vi "Snippets.vi"(6 "args":string[](array[string]), 7 "QD Plugins Dir":path, 8 "error in (no error)":errorcluster, 9 "Shift?":bool, 10 "Focus":enum8{"FP", "BD"}(ring), 11 "VI Refnum":refnum<vi>) -> (0 "error out":errorcluster)   [LabVIEW 2019]
doc: "Imports or exports a VI Snippet (*.png) image programmatically. Import opens a preview dialog to select a VI Snippet (*.png) from the <b>QuickDrop\\plugins\\Snippets</b> directory. Export prompts the user where to save the VI Snippet (*.png). On export, if nothing is selected the entire VI is exported. Otherwise only the selected Block Diagram GObjects are exported.\n\n[SCRIPT]\nimport=Import VI Snippet\nexport=Export VI Snippet"
uses:
  _Snippets/VI Snippet.lvlibp
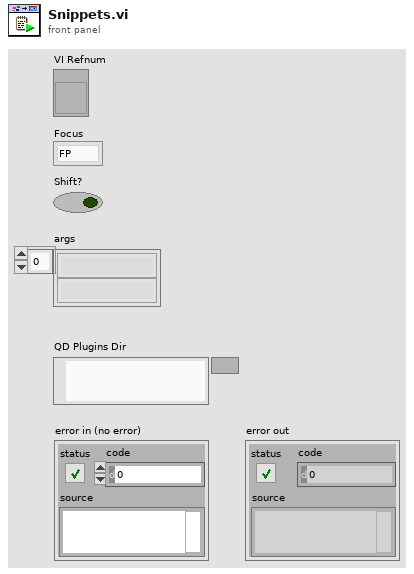
[diagram p1: front panel]
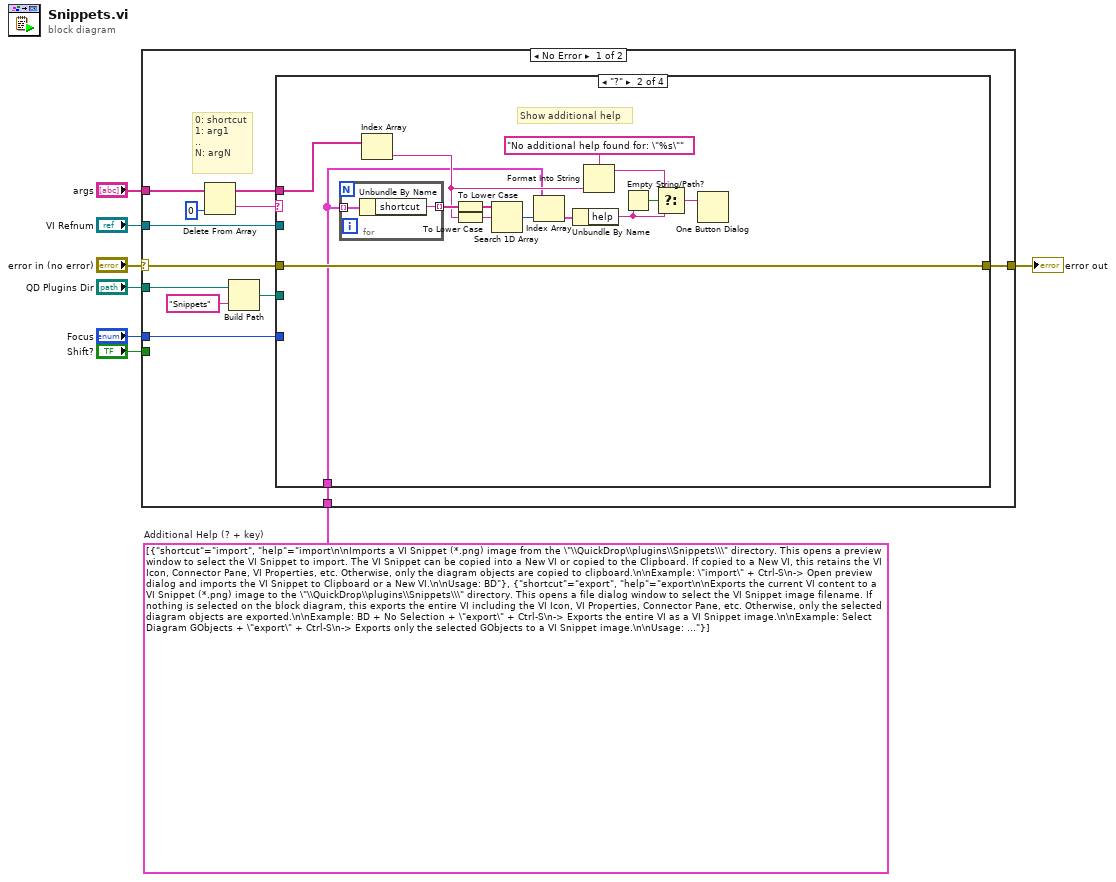
[diagram p0: block diagram]
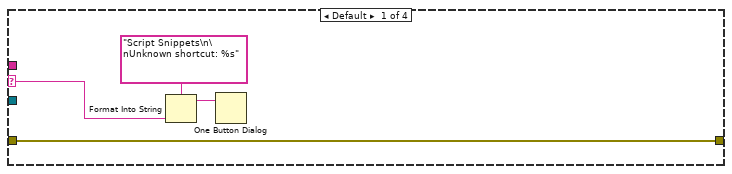
[diagram p2: hidden frame]
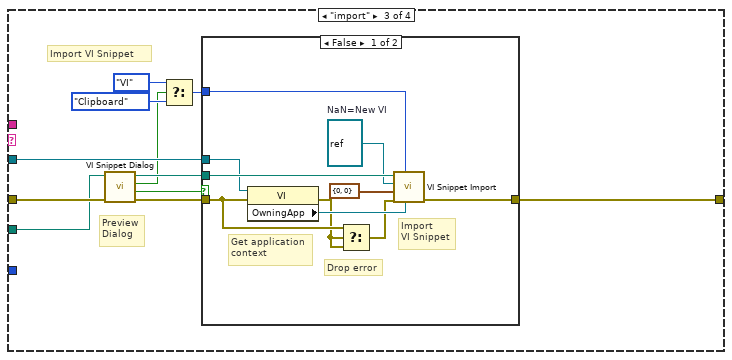
[diagram p3: hidden frame]
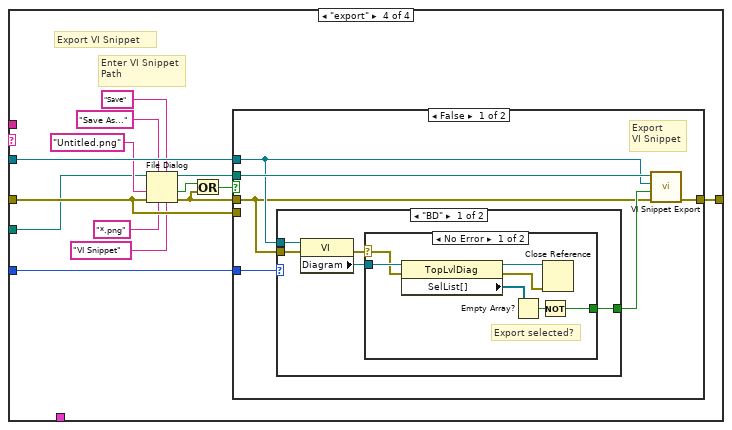
[diagram p5: hidden frame]
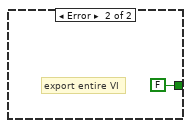
[diagram p6: hidden frame]
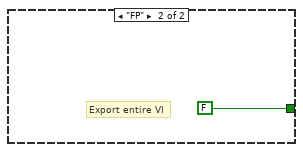
[diagram p7: hidden frame]
diagram:
  w1 = cluster{"shortcut":string, "help":string}[] [{"shortcut"="import", "help"="import\n\nImports a VI Snippet (*.png) image from the \"\\QuickDrop\\plugins\\Snippets\\\" directory. This opens a preview window to select the VI Snippet to import. The VI Snippet can be copied into a New VI or copied to the Clipboard. If copied to a New VI, this retains the VI Icon, Connector Pane, VI Properties, etc. Otherwise, only the diagram objects are copied to clipboard.\n\nExample: \"import\" + Ctrl-S\n-> Open preview dialog and imports the VI Snippet to Clipboard or a New VI.\n\nUsage: BD"}, {"shortcut"="export", "help"="export\n\nExports the current VI content to a VI Snippet (*.png) image to the \"\\QuickDrop\\plugins\\Snippets\\\" directory. This opens a file dialog window to select the VI Snippet image filename. If nothing is selected on the block diagram, this exports the entire VI including the VI Icon, VI Properties, Connector Pane, etc. Otherwise, only the selected diagram objects are exported.\n\nExample: BD + No Selection + \"export\" + Ctrl-S\n-> Exports the entire VI as a VI Snippet image.\n\nExample: Select Diagram GObjects + \"export\" + Ctrl-S\n-> Exports only the selected GObjects to a VI Snippet image.\n\nUsage: BD\n"}]  # Additional Help (? + key)
  n1 = case shown="No Error" "error in (no error)" {
    selector: "error in (no error)" -> [w16 w98]
    tunnel: "VI Refnum" -> [w11 _]
    tunnel: "Focus" -> [w10 _]
    tunnel: "Shift?" -> [_ _]
    tunnel: "args" -> [w19 _]
    tunnel: [w15 w98] -> w3
    tunnel: "QD Plugins Dir" -> [w13 _]
    tunnel: w1 -> [w9 _]
    frame No Error {
      # "0: shortcut\n1: arg1\n..\nN: argN"
      n2 = Delete From Array(array=w19, index=0) -> (deleted portion=w18:string, array with subset deleted=w17:string[])  [unwired: 1 in]
      n3 = Build Path(base path=w13, name or relative path="Snippets") -> (appended path=w14:path)
      n4 = case shown="\"?\"" w18 {
        selector: w18 -> [w21 _ _ _]
        tunnel: [w24 w26 w48 w75] -> w15
        tunnel: w16 -> [w24 w26 w51 w72]
        tunnel: w17 -> [_ w27 _ _]
        tunnel: w14 -> [_ _ w50 w70]
        tunnel: w11 -> [_ _ w46 w74]
        tunnel: w10 -> [_ _ _ w73]
        tunnel: w9 -> [_ w25 _ _]
        frame Default {
          n5 = Format Into String(format string="Script Snippets\n\nUnknown shortcut: %s", w21) -> (resulting string=w22:string)  [unwired: 2 in, 1 out]
          n6 = One Button Dialog(message=w22) -> ()  [unwired: 1 in, 1 out]
        }
        frame "?" {
          # "Show additional help"
          n7 = for {
            tunnel: w25 -> [w40] mode=indexing
            tunnel: [w39] -> w38 mode=indexing
            n8 = Unbundle By Name(w40) -> ("shortcut"=w39:string)
          }
          n9 = Index Array(array=w27) -> (element=w30:string)  [unwired: 1 in]
          n10 = To Lower Case(string=w38) -> (all lower case string=w37:string[])
          n11 = To Lower Case(string=w30) -> (all lower case string=w36:string)
          n12 = Search 1D Array(1D array=w37, element=w36) -> (index of element=w35:i32)  [unwired: 1 in]
          n13 = Index Array(array=w25, index=w35) -> (element=w34:cluster{"shortcut":string, "help":string})
          n14 = Unbundle By Name(w34) -> ("help"=w32:string)
          n15 = Format Into String(format string="No additional help found for: \"%s\"", w30) -> (resulting string=w29:string)  [unwired: 2 in, 1 out]
          n16 = Empty String/Path?(string/path=w32) -> (empty?=w33:bool)
          n17 = Select(t=w29, s=w33, f=w32) -> (s? t:f=w31:string)
          n18 = One Button Dialog(message=w31) -> ()  [unwired: 1 in, 1 out]
        }
        frame "import" {
          # "Import VI Snippet"
          # "Preview\nDialog"
          n19 = call "VI Snippet Dialog.vi"("error in (no error)"=w51, "VI Snippets Dir"=w50) -> ("error out"=w49:errorcluster, "Cancelled?"=w45:bool, "New VI?"=w43:bool, "VI Snippets Path"=w47:path)  [unwired: 6 in]
          n20 = Select(t=enum8{"VI", "Clipboard"}."VI" ("Copy to (\"VI\")"), s=w43, f=enum8{"VI", "Clipboard"}."Clipboard" ("Copy to (\"VI\")")) -> (s? t:f=w41:enum8{"VI", "Clipboard"})
          n21 = case shown="False" w45 {
            tunnel: w49 -> [w55 w62]
            tunnel: [w61 w62] -> w48
            tunnel: w47 -> [w60 _]
            tunnel: w46 -> [w58 _]
            tunnel: w41 -> [w52 _]
            frame False {
              w56 = refnum<vi> refnum  # NaN=New VI
              # "Drop error"
              # "Get application\ncontext"
              # "Import\nVI Snippet"
              n22 = property class="VI"(reference=w58, error in=w55) -> (error out=w54:errorcluster, "OwningApp"=w57:refnum<vi>)  [unwired: 1 out]
              n23 = Select(t=w55, s=w54, f=w54) -> (s? t:f=w53:errorcluster)
              n24 = call "VI Snippet Import.vi"("App Refnum (New VI only)"=w57, "Copy to (\"VI\")"=w52, "error in (no error)"=w53, "Drop Position (0, 0)"=cluster{"Left":i32, "Top":i32} {"Left"=0, "Top"=0}, "VI Refnum in (NaN=New VI)"=w56, "VI Snippet Path (*.png)"=w60) -> ("error out"=w61:errorcluster)  [unwired: 2 in, 3 out]
            }
            frame True {
              # "Cancelled"
            }
          }
        }
        frame "export" {
          # "Export VI Snippet"
          # "Enter VI Snippet\nPath"
          n25 = File Dialog(4:"VI Snippet" ("pattern label"), 5:"Save" ("button label"), 6:"*.png" ("pattern (all files)"), 7:"Save As..." ("prompt"), 8:w72, 9:"Untitled.png" ("default name"), 11:w70) -> (0:w69:errorcluster, 1:w68:bool, 3:w67:path)  [unwired: 1 out]
          n26 = Or(x=w68, y=w69) -> (x .or. y?=w76:bool)
          n27 = case shown="False" w76 {
            tunnel: w72 -> [_ w97]
            tunnel: [w81 w97] -> w75
            tunnel: w67 -> [w82 _]
            tunnel: w69 -> [w77 _]
            tunnel: w74 -> [w78 _]
            tunnel: w73 -> [w79 _]
            frame False {
              # "Export\nVI Snippet"
              n28 = case shown="\"BD\"" w79 {
                tunnel: [w84 FALSE ("Selected GObjects Only? (F)")] -> w80
                tunnel: w78 -> [w87 _]
                tunnel: w77 -> [w83 _]
                frame "BD" {
                  n29 = property class="VI"(reference=w87, error in=w83) -> (error out=w85:errorcluster, "Diagram"=w86:refnum<vi>)  [unwired: 1 out]
                  n30 = case shown="No Error" w85 {
                    selector: w85 -> [w93 _]
                    tunnel: w86 -> [w94 _]
                    tunnel: [w88 FALSE] -> w84
                    frame No Error {
                      # "Export selected?"
                      n31 = property class="TopLvlDiag"(reference=w94, error in=w93) -> (reference out=w91:refnum<vi>, error out=w90:errorcluster, "SelList[]"=w92:refnum<vi>[])
                      n32 = Empty Array?(array=w92) -> (empty?=w89:bool)
                      n33 = Not(x=w89) -> (.not. x?=w88:bool)
                      n34 = Close Reference(reference=w91, error in (no error)=w90) -> ()  [unwired: 1 out]
                    }
                    frame Error {
                      # "export entire VI"
                    }
                  }
                }
                frame "FP" {
                  # "Export entire VI"
                }
              }
              n35 = call "VI Snippet Export.vi"("error in (no error)"=w77, "Selected GObjects Only? (F)"=w80, "VI Refnum"=w78, "VI Snippet Path (*.png)"=w82) -> ("error out"=w81:errorcluster)  [unwired: 7 in]
            }
            frame True {
              # "Cancelled"
            }
          }
        }
      }
    }
    frame Error {
    }
  }
  "error out" <- w3
